vi "read target configuration.vi"(8 "error in":errorcluster, 11 "Targets in":refnum<class "Targets.lvclass">) -> (0 "error out":errorcluster, 2 "Target Configuration":refnum<class "PL_Target Configuration.lvclass">, 3 "Targets out":refnum<class "Targets.lvclass">)   [LabVIEW 2013, in "Targets.lvclass"]
uses:
  Targets.lvclass
  Framework Configuration Classes/target configuration/PL_Target Configuration.lvclass
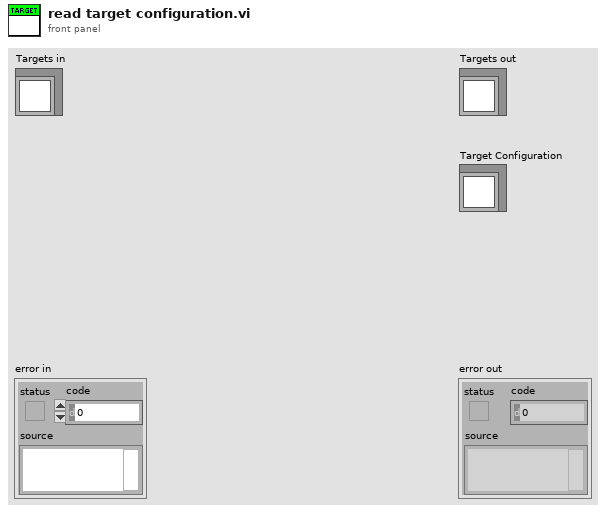
[diagram p1: front panel]
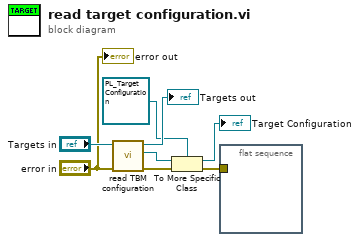
[diagram p0: block diagram]
diagram:
  n1 = call-dynamic "read TBM configuration.vi"("error in"="error in", "TBM Configuration Node in"="Targets in") -> ("error out"=w8:errorcluster, "configuration"=w5:refnum<class "TBM configuration.lvclass">, "TBM Configuration Node out"=→"Targets out":refnum<class "Targets.lvclass">)  [unwired: 7 in]
  n2 = To More Specific Class(target class=refnum<class "PL_Target Configuration.lvclass"> refnum ("Target Configuration"), reference=w5, error in=w8) -> (specific class reference=→"Target Configuration":refnum<class "PL_Target Configuration.lvclass">, error out=w1:errorcluster)
  n3 = flat-sequence {
    tunnel: w1 -> [_]
    frame #0 {
    }
  }
  "error out" <- "error in"
